vi "shoot high goal.vi"(8 "error in (no error)":errorcluster) -> (0 "error out":errorcluster)   [LabVIEW 2015]
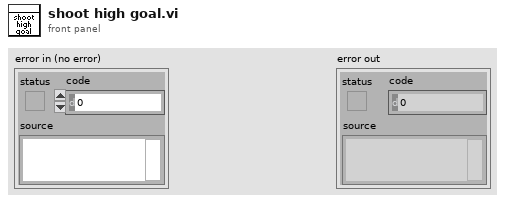
[diagram p1: front panel]
types:
  T1 = typedef "WPI_MotorControlDeviceRef.ctl" = cluster{"DeviceStatus":errorcluster, "Type":T2, "PWM":cluster{"PWM Channel":T3, "DeadBand":T4}, "CAN":cluster{"Device Number":u8, "Control Mode":T5, "Semaphore":T6, "Max Vout":dbl, "TalonSRX Control Mode":T7}, "Invert":bool}
  T2 = typedef "WPI_MotorControlType.ctl" = enum16{"PWM", "CAN", "CANTalonSRX"}
  T3 = typedef "FPGA_DIOPWMChannel.ctl" = enum8{"PWM 0", "PWM 1", "PWM 2", "PWM 3", "PWM 4", "PWM 5", "PWM 6", "PWM 7", "PWM 8", "PWM 9", "PWM MXP 0", "PWM MXP 1", "PWM MXP 2", "PWM MXP 3", "PWM MXP 4", "PWM MXP 5", "PWM MXP 6", "PWM MXP 7", "PWM MXP 8", "PWM MXP 9", "Invalid"}
  T4 = typedef "WPI_PWMDeadband.ctl" = cluster{"Name":string, "maxPositivePwm":i32, "minPositivePwm":i32, "centerPwm":i32, "maxNegativePwm":i32, "minNegativePwm":i32, "angularRange":u16}
  T5 = typedef "WPI_CANJaguar_ControlMode.ctl" = enum8{"Percent VBus", "Current", "Speed", "Position", "Voltage"}
  T6 = typedef "Semaphore RefNum" = refnum<k1>
  T7 = typedef "WPI_CANTalonSRX_APIControlMode.ctl" = enum8{"Percent VBus", "Speed", "Position", "Slave", "Unchanged / Invalid", "Voltage Compensation", "Current", "Motion Profile"}
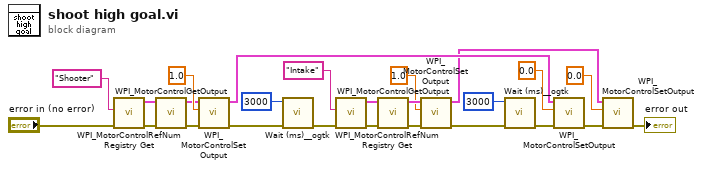
[diagram p0: block diagram]
diagram:
  n1 = call <vilib>:"WPI_MotorControlRefNum Registry Get.vi"("error in (no error)"="error in (no error)", "refnum name"="Shooter") -> ("error out"=w16:errorcluster, "MotorControlDevRef"=w21:T1)  [unwired: 8 in]
  n2 = call <vilib>:"WPI_MotorControlGetOutput.vi"("error in (no error)"=w16, "MotorControlDevRef"=w21) -> ("error out"=w17:errorcluster, "MotorControlDevRef"=w18:T1)  [unwired: 7 in, 1 out]
  n3 = call <vilib>:"WPI_MotorControlSetOutput.vi"("error in (no error)"=w17, "Output"=1.0, "MotorControlDevRef"=w18) -> ("error out"=w13:errorcluster, "MotorControlDevRef"=w8:T1)  [unwired: 6 in, 1 out]
  n4 = call <userlib>:"Wait (ms)__ogtk.vi"("error in (no error)"=w13, "milliseconds to wait"=u32 3000) -> ("error out"=w12:errorcluster)  [unwired: 8 in, 1 out]
  n5 = call <vilib>:"WPI_MotorControlRefNum Registry Get.vi"("error in (no error)"=w12, "refnum name"="Intake") -> ("error out"=w15:errorcluster, "MotorControlDevRef"=w24:T1)  [unwired: 8 in]
  n6 = call <vilib>:"WPI_MotorControlGetOutput.vi"("error in (no error)"=w15, "MotorControlDevRef"=w24) -> ("error out"=w14:errorcluster, "MotorControlDevRef"=w25:T1)  [unwired: 7 in, 1 out]
  n7 = call <vilib>:"WPI_MotorControlSetOutput.vi"("error in (no error)"=w14, "Output"=1.0, "MotorControlDevRef"=w25) -> ("error out"=w9:errorcluster, "MotorControlDevRef"=w7:T1)  [unwired: 6 in, 1 out]
  n8 = call <userlib>:"Wait (ms)__ogtk.vi"("error in (no error)"=w9, "milliseconds to wait"=u32 3000) -> ("error out"=w6:errorcluster)  [unwired: 8 in, 1 out]
  n9 = call <vilib>:"WPI_MotorControlSetOutput.vi"("error in (no error)"=w6, "Output"=0.0, "MotorControlDevRef"=w8) -> ("error out"=w5:errorcluster)  [unwired: 6 in, 2 out]
  n10 = call <vilib>:"WPI_MotorControlSetOutput.vi"("error in (no error)"=w5, "Output"=0.0, "MotorControlDevRef"=w7) -> ("error out"=→"error out":errorcluster)  [unwired: 6 in, 2 out]
